vi "Derivative (single).vi"(6 "Type":enum16{"dy/dx vs x", "dx/dy vs y"}(ring), 8 "error in (no error)":errorcluster, 11 "XY-data":cluster{"X-array":dbl[], "Y-array":dbl[]}) -> (0 "error out":errorcluster, 2 "Differential out":cluster{"X-array":dbl[], "Y-array":dbl[]} {"Y-array" format="%.2p"; "X-array" format="%.2p"}, 3 "XY-data out":cluster{"X-array":dbl[], "Y-array":dbl[]})   [LabVIEW 2019, in "xy_utilities.lvlib"]
doc: "Performs numerical differentiation of <b>XY-data</b> using the finite difference method.\n\n<b>Interval</b> is the range over which the finite difference is calculated.\n<b>Interval Units</b> defines the units of the <b>Interval</b> to be the number of points or the same units as the x (or y) data.\n<b>Type</b> specifies taking a derivative with respect to x or y.\n\nWire data to the data input to determine the polymorphic instance to use or manually select the instance."
uses:
  xy_utilities.lvlib
  <vilib>/Analysis/NI_AALPro.lvlib
  Swap X and Y (single).vi
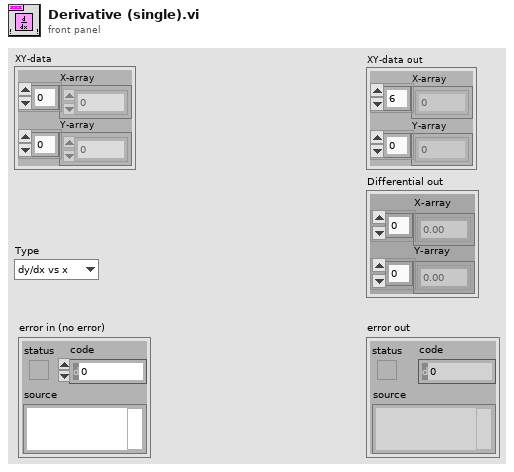
[diagram p1: front panel]
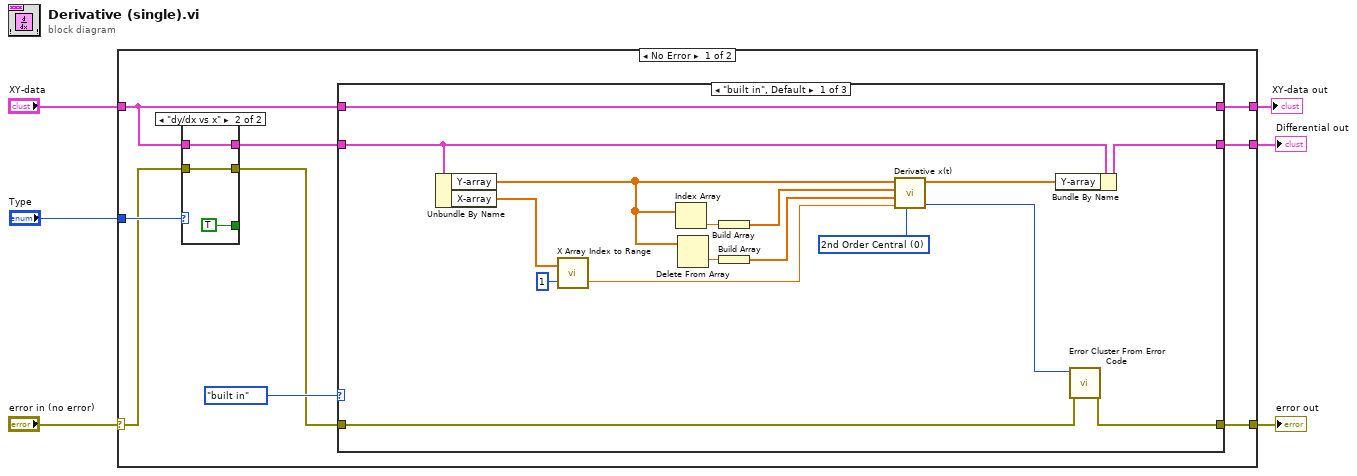
[diagram p0: block diagram]
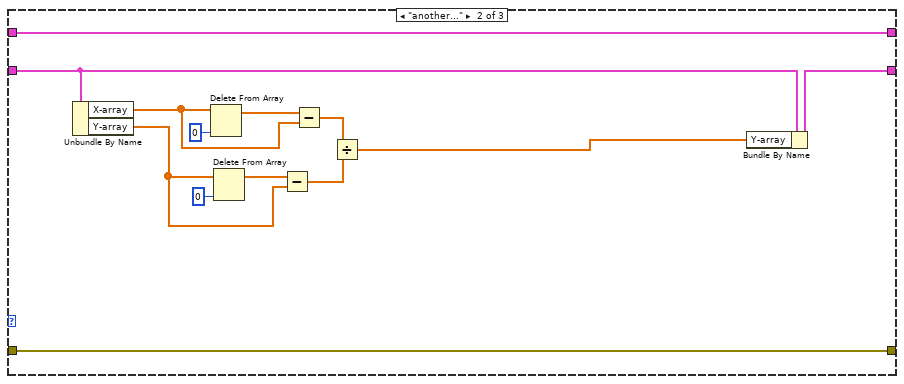
[diagram p2: hidden frame]
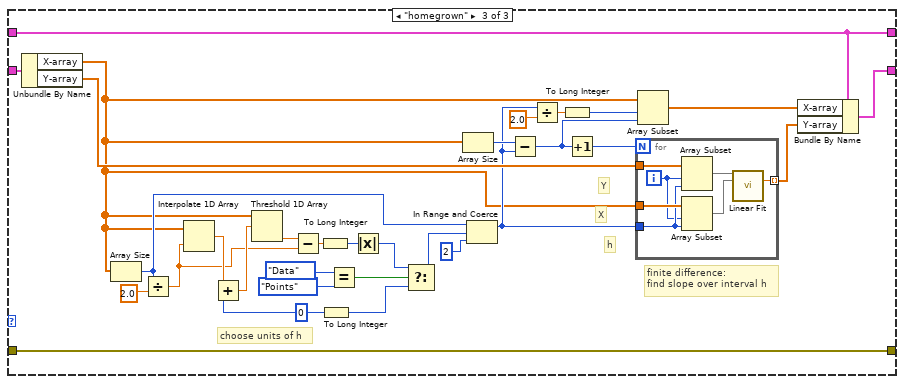
[diagram p3: hidden frame]
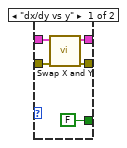
[diagram p4: hidden frame]
diagram:
  n1 = case shown="No Error" "error in (no error)" {
    selector: "error in (no error)" -> [w14 w92]
    tunnel: [w9 w92] -> w5
    tunnel: "XY-data" -> [w13 w91]
    tunnel: [w12 _] -> w3
    tunnel: "Type" -> [w15 _]
    tunnel: [w10 w91] -> w1
    frame No Error {
      n2 = case shown="\"dy/dx vs x\"" w15 {
        tunnel: w13 -> [w87 w90]
        tunnel: [w86 w90] -> w11
        tunnel: [w85 w89] -> w7
        tunnel: w14 -> [w84 w89]
        tunnel: [FALSE ("dy/dx vs x") TRUE ("dy/dx vs x")] -> _
        frame "dx/dy vs y" {
          n3 = call-poly "Swap X and Y.vi"("error in (no error)"=w84, "XY-data"=w87) -> ("error out"=w85:errorcluster, "XY-data out"=w86:cluster{"X-array":dbl[], "Y-array":dbl[]})  [unwired: 8 in]
        }
        frame "dy/dx vs x" {
        }
      }
      n4 = case shown="\"built in\", Default" enum16{"built in", "another...", "homegrown"}."built in" ("Subset Method") {
        tunnel: w13 -> [w27 w43 w57]
        tunnel: [w21 w35 w63] -> w12
        tunnel: w11 -> [w28 w37 w45]
        tunnel: [w27 w43 w57] -> w10
        tunnel: [w29 w44 w56] -> w9
        tunnel: w7 -> [w30 w44 w56]
        frame "built in", Default {
          w25 = u16 0 items=["2nd Order Central", "4th Order Central", "Forward", "Backward"] ("method")
          n5 = Unbundle By Name(w28) -> ("Y-array"=w19:dbl[], "X-array"=w18:dbl[])
          n6 = call "X Array Index to Range.vi"("X Range (index)"=1, "X-array"=w18) -> ("X Range"=w16:dbl)  [unwired: 1 in]
          n7 = Index Array(array=w19) -> (element=w24:dbl)  [unwired: 1 in]
          n8 = Delete From Array(array=w19) -> (deleted portion=w20:dbl)  [unwired: 2 in, 1 out]
          n9 = Build Array(w24) -> (w23:dbl[])
          n10 = Build Array(w20) -> (w22:dbl[])
          n11 = call <vilib>:"Derivative x(t).vi"("method"=w25, "dt"=w16, "Final Condition"=w22, "Initial Condition"=w23, "X"=w19) -> ("error"=w31:i32, "dX/dt"=w26:dbl[])  [unwired: 5 in]
          n12 = Bundle By Name(cluster=w28, "Y-array"=w26) -> (w21:cluster{"X-array":dbl[], "Y-array":dbl[]})
          n13 = call <vilib>:"Error Cluster From Error Code.vi"("error in (no error)"=w30, "error code (0)"=w31) -> ("error out"=w29:errorcluster)  [unwired: 7 in]
        }
        frame "another..." {
          n14 = Unbundle By Name(w37) -> ("X-array"=w32:dbl[], "Y-array"=w40:dbl[])
          n15 = Delete From Array(array=w32, index=0) -> (array with subset deleted=w42:dbl[])  [unwired: 1 in, 1 out]
          n16 = Delete From Array(array=w40, index=0) -> (array with subset deleted=w41:dbl[])  [unwired: 1 in, 1 out]
          n17 = Subtract(x=w41, y=w40) -> (x-y=w38:dbl[])
          n18 = Subtract(x=w42, y=w32) -> (x-y=w39:dbl[])
          n19 = Divide(x=w39, y=w38) -> (x/y=w36:dbl[])
          n20 = Bundle By Name(cluster=w37, "Y-array"=w36) -> (w35:cluster{"X-array":dbl[], "Y-array":dbl[]})
        }
        frame "homegrown" {
          w46 = 0 ("number")
          # "choose units of h"
          # "h"
          # "finite difference:\nfind slope over interval h"
          # "Y"
          # "X"
          n21 = Unbundle By Name(w45) -> ("X-array"=w48:dbl[], "Y-array"=w58:dbl[])
          n22 = Array Size(array=w48) -> (size(s)=w55:i32)
          n23 = Divide(x=w55, y=2.0) -> (x/y=w49:dbl)
          n24 = Interpolate 1D Array(1:w49, 2:w48) -> (0:w50:dbl)
          n25 = Add(x=w50, y=w46) -> (x+y=w65:dbl)
          n26 = Threshold 1D Array(2:w65, 3:w48) -> (0:w67:dbl)  [unwired: 1 in]
          n27 = Subtract(x=w67, y=w49) -> (x-y=w66:dbl)
          n28 = To Long Integer(number=w66) -> (32bit integer=w64:i32)
          n29 = To Long Integer(number=w46) -> (32bit integer=w60:i32)
          n30 = Equal?(x=enum16{"Points", "Data"}."Data" ("Interval Units"), y=enum16{"Points", "Data"}."Points") -> (x = y?=w61:bool)
          n31 = Absolute Value(x=w64) -> (abs(x)=w53:i32)
          n32 = Select(t=w53, s=w61, f=w60) -> (s? t:f=w52:i32)
          n33 = Array Size(array=w48) -> (size(s)=w71:i32)
          n34 = In Range and Coerce(upper limit=w55, x=w52, lower limit=2) -> (coerced(x)=w51:i32)  [unwired: 1 out]
          n35 = Subtract(x=w71, y=w51) -> (x-y=w74:i32)
          n36 = Divide(x=w51, y=2.0) -> (x/y=w69:dbl)
          n37 = To Long Integer(number=w69) -> (32bit integer=w75:i32)
          n38 = Increment(x=w74) -> (x+1=w72:i32)
          n39 = for {
            N: w72 -> [_]
            tunnel: w58 -> [w82]
            tunnel: w48 -> [w81]
            tunnel: w51 -> [w80]
            tunnel: [w79] -> w59 mode=indexing
            i -> [w76]
            n40 = Array Subset "Array Subset"(array=w82, index=w76, length=w80) -> (w78:dbl[])
            n41 = Array Subset(array=w81, index=w76, length=w80) -> (w77:dbl[])
            n42 = call <vilib>:"Linear Fit.vi"("Y"=w78, "X"=w77) -> ("slope"=w79:dbl)  [unwired: 9 in, 4 out]
          }
          n43 = Array Subset(array=w48, index=w75, length=w74) -> (w73:dbl[])
          n44 = Bundle By Name(cluster=w57, "X-array"=w73, "Y-array"=w59) -> (w63:cluster{"X-array":dbl[], "Y-array":dbl[]})
        }
      }
    }
    frame Error {
    }
  }
  "error out" <- w5
  "Differential out" <- w3
  "XY-data out" <- w1
